vi "ImageAcquisition_test.vi"(0 "Log Image":bool=TRUE, 4 "Number of Image Buffers":u32=10, 5 "Stop (F)":bool, 7 "error in":errorcluster) -> (20 "Image Out":T2(plugin-control), 21 "All Image Buffers Out":T2[](array[typedef]), 22 "Image Number":u32, 23 "Lost Image Count":u32, 24 "Total Images Transferred":u32, 25 "Frame Rate":dbl, 26 "Stopped":bool, 27 "error out":errorcluster)   [LabVIEW 2018]
doc: "Creates, and edits acquisitions using the NI Vision Acquisition Express VI.\n\nThe NI Vision Acquisition Wizard is launched by placing the Express VI on the block diagram. Select an acquisition source and configure an acquisition using NI-IMAQ, NI-IMAQdx, or simulate an acquisition by reading an AVI or image files from a folder. After an acquisition is configured, select controls and indicators to be able to programmatically set in LabVIEW. Double-click the Vision Acquisition Express VI to edit the acquisition.\n\nNote: Any images created by the Express VI need to be disposed after use. Use the IMAQ Dispose.vi to cleanup the images output by the Express VI when they are no longer needed."
uses:
  <vilib>/vision/Image Controls.llb/IMAQ Image.ctl
  <vilib>/vision/driver/IMAQdx.llb/IMAQdx Buffer Number Mode.ctl
  <vilib>/vision/driver/IMAQdx.llb/IMAQdx Acquisition Mode.ctl
  <vilib>/vision/driver/Vision Acquisition Express Utility VIs.llb/Vision Acquisition Path Convert (String).vi
  <vilib>/vision/driver/NI_Vision_Acquisition_Software.lvlib
  <resource>/objmgr/imaqdx.rc
panel:
  in  "Origin 2":cluster{"X":i32, "Y":i32}={"X"=1120, "Y"=715}
  in  "Text Color":u32(colorbox)=16777226
  in  "Origin":cluster{"X":i32, "Y":i32}={"X"=1120, "Y"=680}
  in  "Font, Size & Style":T1={"Desired Font (Application)"=enum."User-specified Font", "[User-specified Font]"={"Font Name"="", "Size"=35, "Strikeout?"=FALSE, "Italic?"=FALSE, "Underline?"=FALSE, "Outline?"=FALSE, "Shadow?"=FALSE, "Bold?"=TRUE, "Rotation Angle"=0.0}, "Horizontal Alignment"=0, "Vertical Alignment"=0} {"Vertical Alignment" items=["Bottom", "Top", "Baseline"]; "Horizontal Alignment" items=["Left", "Center", "Right"]; "[User-specified Font]"."Rotation Angle" format="%.2f"}
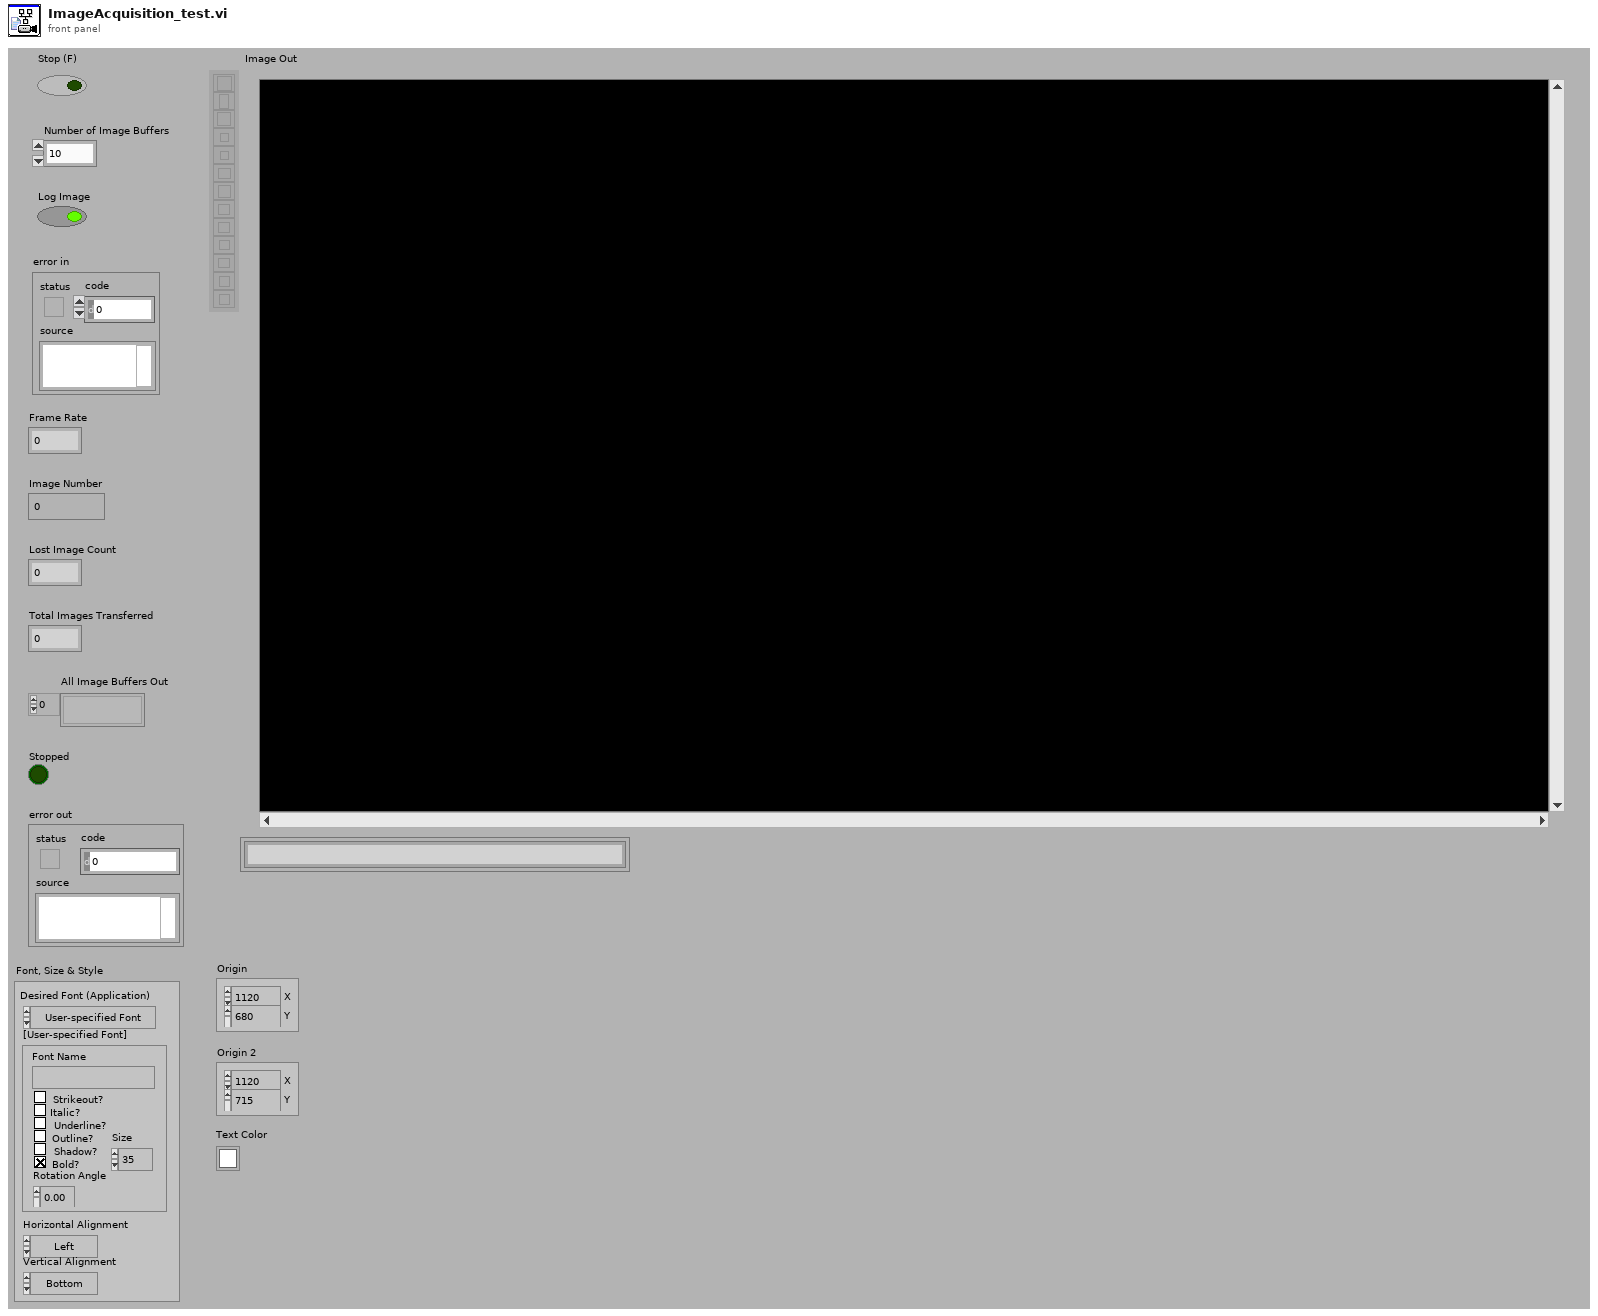
[diagram p1: front panel]
types:
  T1 = cluster{"Desired Font (Application)":enum16{"User-specified Font", "Application Font", "System Font", "Dialog Font"}, "[User-specified Font]":cluster{"Font Name":string, "Size":i16, "Strikeout?":bool, "Italic?":bool, "Underline?":bool, "Outline?":bool, "Shadow?":bool, "Bold?":bool, "Rotation Angle":dbl}, "Horizontal Alignment":i16, "Vertical Alignment":i16}
  T2 = typedef "IMAQ Image.ctl" = refnum<image>
  T3 = typedef "NI_Vision_Acquisition_Software.lvlib/IMAQdx Buffer Number Mode.ctl" = enum32{"Next", "Last", "Buffer Number", "Every", "Last New"}
  T4 = typedef "NI_Vision_Acquisition_Software.lvlib/IMAQdx Acquisition Mode.ctl" = enum32{"One Shot", "Continuous"}
  T5 = typedef "IMAQdx.ctl" = refnum<k21>
  T6 = cluster{"File Type":string, "Quality":u32, "Compress":bool, "Lossless":bool, "Ratio":sgl, "Codec":string, "Frame Rate":u32, "Limit Frames":bool, "Max Frames":u32}
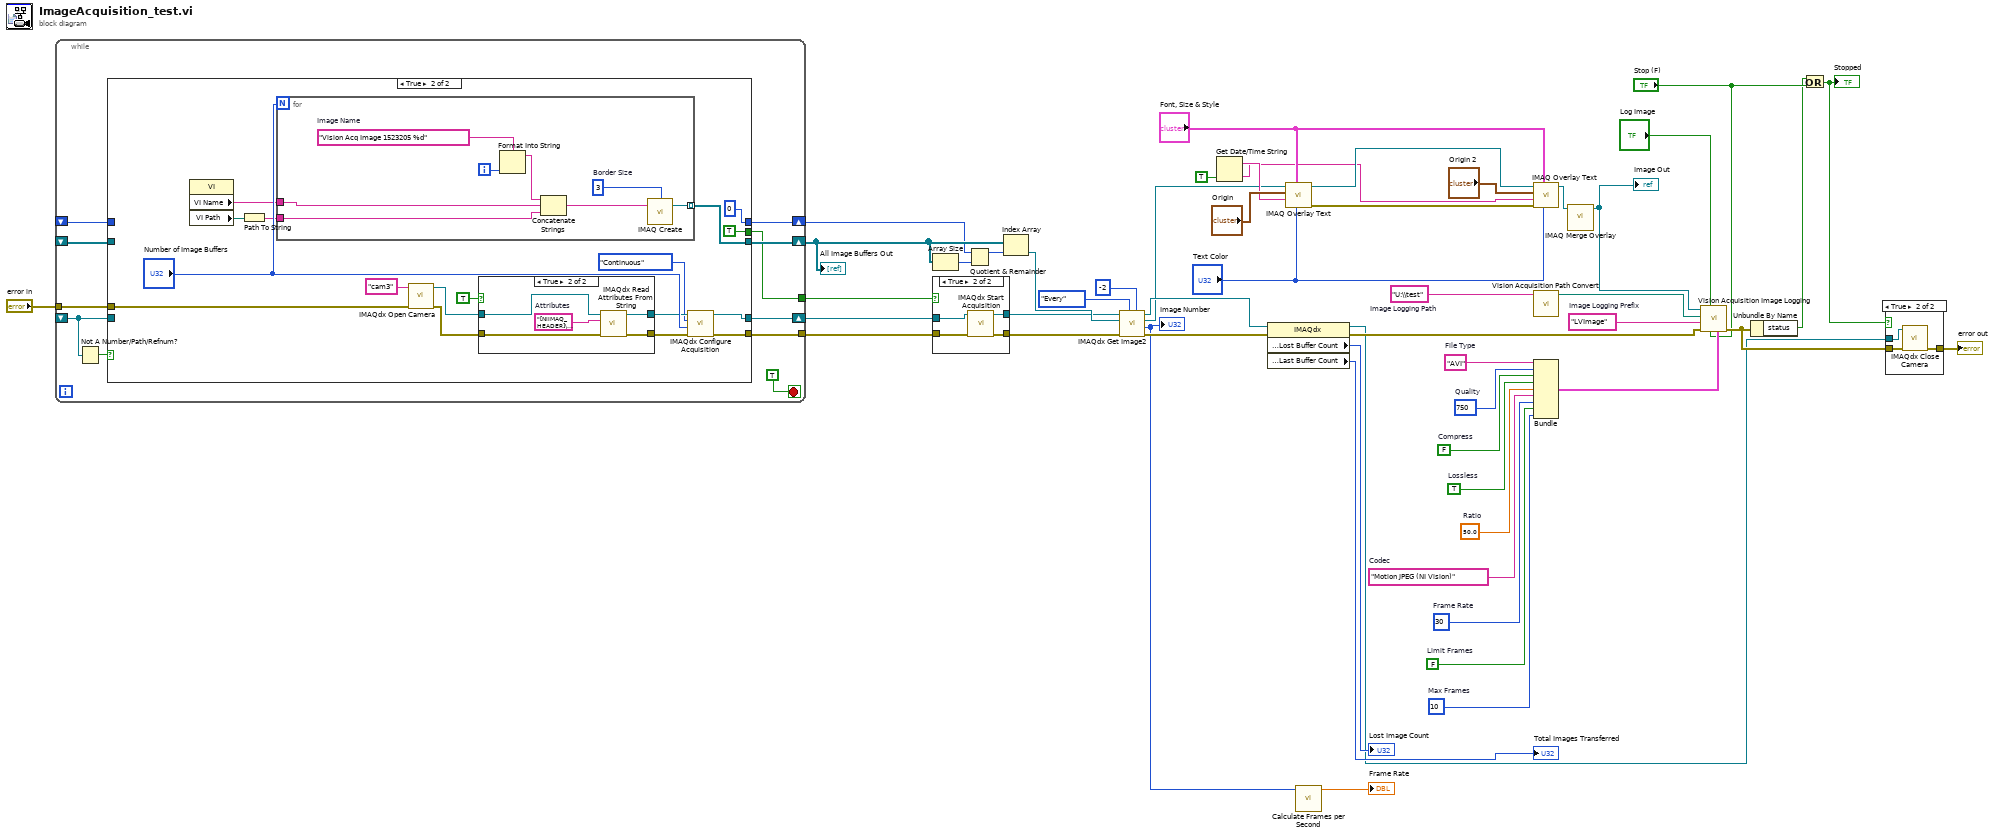
[diagram p0: block diagram]
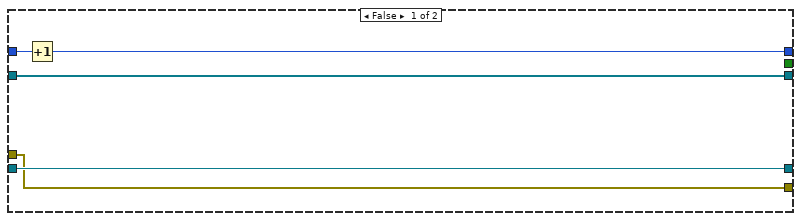
[diagram p4: hidden frame]
diagram:
  w18 = "U:\\test"  # Image Logging Path
  w32 = "LVImage"  # Image Logging Prefix
  w27 = sgl 50.0  # Ratio
  w28 = TRUE  # Lossless
  w29 = FALSE  # Compress
  w30 = u32 750  # Quality
  w26 = "Motion JPEG (NI Vision)"  # Codec
  w25 = u32 30  # Frame Rate
  w23 = u32 10  # Max Frames
  w24 = FALSE  # Limit Frames
  w31 = "AVI"  # File Type
  n1 = while {
    shift-right: [w63] -> w41
    shift-left: _ -> [w55]
    tunnel: [w62] -> w51
    tunnel: "error in" -> [w61]
    shift-right: [w59] -> w45
    shift-left: _ -> [w58]
    shift-right: [w57] -> w38
    shift-left: _ -> [w56]
    tunnel: [w53] -> w37
    stop <- TRUE stop-if-true
    n2 = Not A Number/Path/Refnum?(number/path/refnum=w55) -> (NaN/Path/Refnum?=w54:bool)
    n3 = case shown="True" w54 {
      tunnel: [w68 w83] -> w63
      tunnel: w55 -> [w68 _]
      tunnel: [w67 w82] -> w62
      tunnel: w61 -> [w67 w85]
      tunnel: [w66 w81] -> w59
      tunnel: w58 -> [w66 _]
      tunnel: [w64 0] -> w57
      tunnel: w56 -> [w65 _]
      tunnel: [_ TRUE] -> w53
      frame False {
        n4 = Increment(x=w65) -> (x+1=w64:i32)
      }
      frame True {
        n5 = property class="VI"() -> ("VI Name"=w77:string, "VI Path"=w78:path)  [unwired: 2 in, 2 out]
        n6 = Path To String(path=w78) -> (string=w76:string)
        n7 = for "For Loop_template0" {
          N: "Number of Image Buffers" -> [_]
          tunnel: [w100] -> w81 mode=indexing
          tunnel: w77 -> [w95]
          tunnel: w76 -> [w94]
          i -> [w99]
          w93 = 3  # Border Size
          w98 = "Vision Acq Image 1523205 %d"  # Image Name
          n8 = Format Into String(format string=w98, w99) -> (resulting string=w97:string)  [unwired: 2 in, 1 out]
          n9 = Concatenate Strings(w97, w95, w94) -> (w96:string)
          n10 = call "IMAQ Create"("Border Size"=w93, "Image Name"=w96) -> ("New Image"=w100:T2)  [unwired: 2 in, 2 out]
        }
        n11 = call <vilib>:"IMAQdx Open Camera.vi"("error in"=w85, "Session In"="cam3" ("Interface Name")) -> ("error out"=w74:errorcluster, "Session Out"=w75:T5)  [unwired: 1 in, 7 out]
        n12 = case shown="True" TRUE ("Init Attributes") {
          tunnel: w75 -> [w87 w92]
          tunnel: w74 -> [w86 w91]
          tunnel: [w87 w89] -> w73
          tunnel: [w86 w88] -> w72
          frame False {
          }
          frame True {
            w90 = "[NIIMAQ_HEADER]\nType = 2\nVersion = 8\n\n[CAMERA_DATA]\nAcquisitionAttributes::Bayer::Algorithm = \"Bilinear\"\nAcquisitionAttributes::Bayer::GainB = \"1\"\nAcquisitionAttributes::Bayer::GainG = \"1\"\nAcquisitionAttributes::Bayer::GainR = \"1\"\nAcquisitionAttributes::Bayer::Pattern = \"Use hardware value\"\nAcquisitionAttributes::BitsPerPixel = \"Use hardware value\"\nAcquisitionAttributes::HardwareMaximumQueuedBufferCount = \"1000\"\nAcquisitionAttributes::HardwareRequeueBufferListThreshold = \"50\"\nAcquisitionAttributes::IgnoreFirstFrame = \"false\"\nAcquisitionAttributes::ImageDecoderCopyMode = \"Auto\"\nAcquisitionAttributes::OutputImageType = \"Auto\"\nAcquisitionAttributes::OverwriteMode = \"Get Newest\"\nAcquisitionAttributes::PixelSignedness = \"Use hardware value\"\nAcquisitionAttributes::ReceiveTimestampMode = \"None\"\nAcquisitionAttributes::ShiftPixelBits = \"false\"\nAcquisitionAttributes::SwapPixelBytes = \"false\"\nAcquisitionAttributes::Timeout = \"5000\"\nAcquisitionAttributes::VerticalMirror = \"false\"\nAcquisitionAttributes::VideoMode = \"1280x720 MJPG 30.00fps\"\nCameraAttributes::BacklightCompensation::Mode = \"Manual\"\nCameraAttributes::BacklightCompensation::Value = \"false\"\nCameraAttributes::Brightness::Mode = \"Manual\"\nCameraAttributes::Brightness::Value = \"128\"\nCameraAttributes::Contrast::Mode = \"Manual\"\nCameraAttributes::Contrast::Value = \"1.28\"\nCameraAttributes::Exposure::Mode = \"Auto\"\nCameraAttributes::Focus::Mode = \"Auto\"\nCameraAttributes::Gain::Mode = \"Manual\"\nCameraAttributes::Gain::Value = \"77\"\nCameraAttributes::Pan::Mode = \"Manual\"\nCameraAttributes::Pan::Value = \"0\"\nCameraAttributes::Saturation::Mode = \"Manual\"\nCameraAttributes::Saturation::Value = \"128\"\nCameraAttributes::Sharpness::Mode = \"Manual\"\nCameraAttributes::Sharpness::Value = \"128\"\nCameraAttributes::Tilt::Mode = \"Manual\"\nCameraAttributes::Tilt::Value = \"0\"\nCameraAttributes::WhiteBalance::Mode = \"Auto\"\nCameraAttributes::Zoom::Mode = \"Manual\"\nCameraAttributes::Zoom::Value = \"100\"\n"  # Attributes
            n13 = call <vilib>:"IMAQdx Read Attributes From String.vi"("error in"=w91, "Attributes String In"=w90, "Session In"=w92) -> ("error out"=w88:errorcluster, "Session Out"=w89:T5)  [unwired: 7 out]
          }
        }
        n14 = call <vilib>:"IMAQdx Configure Acquisition.vi"("error in"=w72, "Number of Buffers"="Number of Image Buffers", "Continuous?"=IMAQdx_Acquisition_Mode."Continuous", "Session In"=w73) -> ("error out"=w82:errorcluster, "Session Out"=w83:T5)  [unwired: 6 out]
      }
    }
  }
  "All Image Buffers Out" <- w45
  n15 = Array Size(array=w45) -> (size(s)=w46:i32)
  n16 = case shown="True" w37 {
    tunnel: w41 -> [w102 w106]
    tunnel: w51 -> [w101 w105]
    tunnel: [w101 w104] -> w39
    tunnel: [w102 w103] -> w40
    frame False {
    }
    frame True {
      n17 = call <vilib>:"IMAQdx Start Acquisition.vi"("error in"=w105, "Session In"=w106) -> ("error out"=w104:errorcluster, "Session Out"=w103:T5)  [unwired: 8 out]
    }
  }
  n18 = Quotient & Remainder(x=w38, y=w46) -> (x-y*floor(x/y)=w44:i32)  [unwired: 1 out]
  n19 = Index Array(array=w45, index=w44) -> (element=w43:T2)
  n20 = call <vilib>:"IMAQdx Get Image2.vi"("Timeout (ms)"=-2, "Buffer Number Mode (Next)"=IMAQdx_Buffer_Number_Mode."Every", "error in"=w39, "Image In"=w43, "Session In"=w40) -> ("error out"=w49:errorcluster, "Buffer Number Out"=w36:u32, "Image Out"=w3:T2, "Session Out"=w50:T5)  [unwired: 3 in]
  "Image Number" <- w36
  n21 = Get Date/Time String(want seconds? (F)=TRUE) -> (date string=w11:string, time string=w6:string)  [unwired: 2 in]
  n22 = property class="IMAQdx"(reference=w50, error in=w49) -> (reference out=w17:T5, error out=w42:errorcluster, "Status Information:Lost Buffer Count"=→"Lost Image Count":u32, "Status Information:Last Buffer Count"=→"Total Images Transferred":u32)
  n23 = call "IMAQ Overlay Text"("Text Color (black)"="Text Color", "Font, Size & Style"="Font, Size & Style", "String"=w11, "Origin"="Origin", "Image"=w3) -> ("error out"=w10:errorcluster, "Image Out"=w9:T2)  [unwired: 5 in]
  n24 = call <vilib>:"Calculate Frames per Second.vi"("Buffer Number"=w36) -> ("Acquired Frames/s"=→"Frame Rate":dbl)  [unwired: 2 in, 8 out]
  n25 = call "IMAQ Overlay Text"("Text Color (black)"="Text Color", "Font, Size & Style"="Font, Size & Style", "error in (no error)"=w10, "String"=w6, "Origin"="Origin 2", "Image"=w9) -> ("Image Out"=w2:T2)  [unwired: 4 in, 1 out]
  n26 = call-poly <vilib>:"Vision Acquisition Path Convert.vi"("Path In"=w18) -> ("Path Out"=w19:path)  [unwired: 10 in]
  n27 = Bundle("File Type"=w31, "Quality"=w30, "Compress"=w29, "Lossless"=w28, "Ratio"=w27, "Codec"=w26, "Frame Rate"=w25, "Limit Frames"=w24, "Max Frames"=w23) -> (w20:T6)  [unwired: 1 out]
  n28 = call "IMAQ Merge Overlay"("Image Src"=w2) -> ("Image Dst Out"=w1:T2)  [unwired: 9 in, 1 out]
  "Image Out" <- w1
  n29 = call <vilib>:"Vision Acquisition Image Logging.vi"("File Settings"=w20, "Close"="Stop (F)", "Log Image"="Log Image", "error in (no error)"=w42, "Image Logging Prefix"=w32, "Image Logging Path"=w19, "Image In"=w1) -> ("error out"=w22:errorcluster)  [unwired: 4 out]
  n30 = Unbundle By Name(w22) -> ("status"=w13:bool)
  n31 = Or(x=w13, y="Stop (F)") -> (x .or. y?=w14:bool)
  "Stopped" <- w14
  n32 = case "Case Structure_template1" shown="True" w14 {
    tunnel: [w107 w109] -> w16
    tunnel: w22 -> [w107 w110]
    tunnel: w17 -> [_ w108]
    frame False {
    }
    frame True {
      n33 = call <vilib>:"IMAQdx Close Camera.vi"("error in"=w110, "Session In"=w108) -> ("error out"=w109:errorcluster)  [unwired: 9 out]
    }
  }
  "error out" <- w16
